vi "数据导出Excel.vi"(8 "error in (no error)":errorcluster caption="错误输入（无错误）", 10 "text data":string[][](array[string]) caption="文本数据", 11 "default name":string="历史数据" caption="默认名称") -> (0 "error out":errorcluster caption="错误输出", 3 "布尔":bool)   [LabVIEW 2016]
uses:
  <vilib>/Utility/NIReport.llb/Append Text Table to Report (wrap).vi
  <vilib>/Utility/NIReport.llb/NI_report.lvclass
  <vilib>/Utility/NIReport.llb/Excel/NI_Excel.lvclass
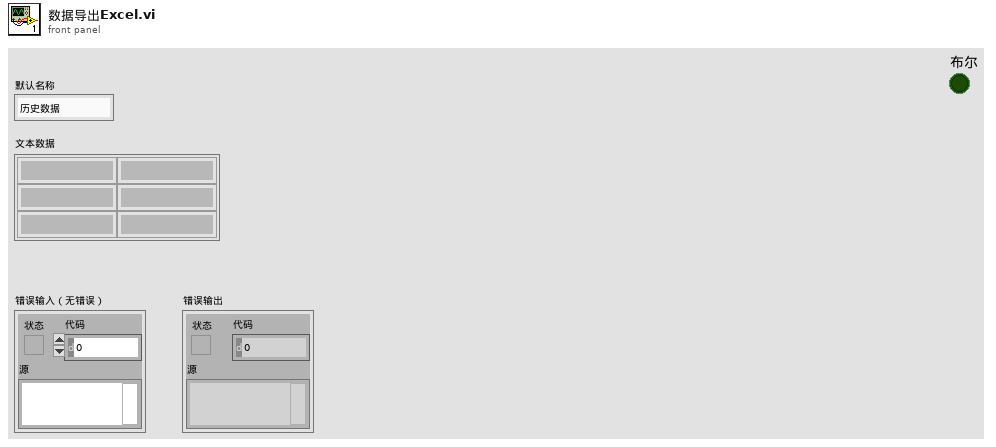
[diagram p1: front panel]
types:
  T1 = enum16{"maximized", "minimized", "normal", "no change"}
  T2 = enum16{"Standard Report", "HTML", "Word", "Excel"}
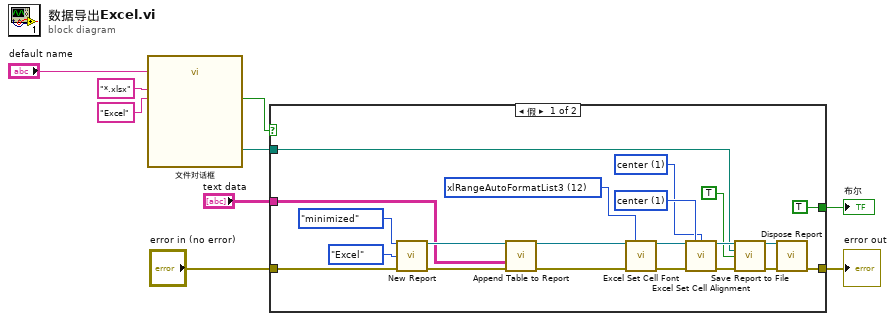
[diagram p0: block diagram]
diagram:
  n1 = call "文件对话框"("default name"="default name", "pattern (all files)"="*.xlsx", "pattern label"="Excel") -> ("selected path"=w6:path, "cancelled"=w7:bool)  [unwired: 9 in, 2 out]
  n2 = case shown="假" w7 {
    tunnel: w6 -> [w15 _]
    tunnel: "error in (no error)" -> [w14 w31]
    tunnel: [w13 w31] -> w4
    tunnel: "text data" -> [w11 _]
    tunnel: [TRUE _] -> w1
    frame False {
      w16 = 1 items=["left", "center", "right"] ("horizontal alignment (left)")
      w17 = 1 items=["top", "center", "bottom"] ("vertical alignment (top)")
      w20 = 12 items=["xlRangeAutoFormat3DEffects1"=13, "xlRangeAutoFormat3DEffects2"=14, "xlRangeAutoFormatAccounting1"=4, "xlRangeAutoFormatAccounting2"=5, "xlRangeAutoFormatAccounting3"=6, "xlRangeAutoFormatAccounting4"=17, "xlRangeAutoFormatClassic1"=1, "xlRangeAutoFormatClassic2"=2, "xlRangeAutoFormatClassic3"=3, "xlRangeAutoFormatColor1"=7, "xlRangeAutoFormatColor2"=8, "xlRangeAutoFormatColor3"=9, "xlRangeAutoFormatList1"=10, "xlRangeAutoFormatList2"=11, "xlRangeAutoFormatList3"=12, "xlRangeAutoFormatLocalFormat1"=15, "xlRangeAutoFormatLocalFormat2"=16, "xlRangeAutoFormatLocalFormat3"=19, "xlRangeAutoFormatLocalFormat4"=20, "xlRangeAutoFormatReport1"=21, "xlRangeAutoFormatReport2"=22, "xlRangeAutoFormatReport3"=23, "xlRangeAutoFormatReport4"=24, "xlRangeAutoFormatReport5"=25, "xlRangeAutoFormatReport6"=26, "xlRangeAutoFormatReport7"=27, "xlRangeAutoFormatReport8"=28, "xlRangeAutoFormatReport9"=29, "xlRangeAutoFormatReport10"=30, "xlRangeAutoFormatClassicPivotTable"=31, "xlRangeAutoFormatTable1"=32, "xlRangeAutoFormatTable2"=33, "xlRangeAutoFormatTable3"=34, "xlRangeAutoFormatTable4"=35, "xlRangeAutoFormatTable5"=36, "xlRangeAutoFormatTable6"=37, "xlRangeAutoFormatTable7"=38, "xlRangeAutoFormatTable8"=39, "xlRangeAutoFormatTable9"=40, "xlRangeAutoFormatTable10"=41, "xlRangeAutoFormatPTNone"=42, "xlRangeAutoFormatNone"=-4142, "xlRangeAutoFormatSimple"=-4154] ("auto format")
      n3 = call <vilib>:"New Report.vi"("window state (normal)"=T1."minimized", "report type"=T2."Excel", "error in (no error)"=w14) -> ("report out"=w26:refnum<class "NI_report.lvclass">, "error out"=w25:errorcluster)  [unwired: 11 in]
      n4 = call-poly <vilib>:"Append Table to Report.vi"("report in"=w26, "text data"=w11, "error in (no error)"=w25) -> ("report out"=w24:refnum<class "NI_report.lvclass">, "error out"=w23:errorcluster)  [unwired: 9 in, 2 out]
      n5 = call <vilib>:"Excel Set Cell Font.vi"("report in"=w24, "auto format"=w20, "error in (no error)"=w23) -> ("report out"=w19:refnum<class "NI_report.lvclass">, "error out"=w18:errorcluster)  [unwired: 11 in]
      n6 = call <vilib>:"Excel Set Cell Alignment.vi"("report in"=w19, "vertical alignment (top)"=w17, "horizontal alignment (left)"=w16, "error in (no error)"=w18) -> ("report out"=w22:refnum<class "NI_report.lvclass">, "error out"=w21:errorcluster)  [unwired: 10 in]
      n7 = call-dynamic "Save Report to File.vi"("report in"=w22, "report file path"=w15, "prompt to replace? (F)"=TRUE, "error in (no error)"=w21) -> ("report out"=w28:refnum<class "NI_report.lvclass">, "error out"=w27:errorcluster)  [unwired: 10 in]
      n8 = call-dynamic "Dispose Report.vi"("report in"=w28, "error in (no error)"=w27) -> ("error out"=w13:errorcluster)  [unwired: 13 in]
    }
    frame True {
    }
  }
  "error out" <- w4
  "布尔" <- w1
